vi "Test Constant Waveform Iterate Functions.vi"() -> ()   [LabVIEW 2021]
uses:
  <vilib>/measure/NI_MABase.lvlib
  Source/Constants/Support/WFM/WFM.vi
  Source/Constants/Support/WFM/Const_WFM.lvclass
panel:
  out "Waveform Chart 2":waveform(dbl)(graph)
  out "Waveform Chart":waveform(dbl)(graph)
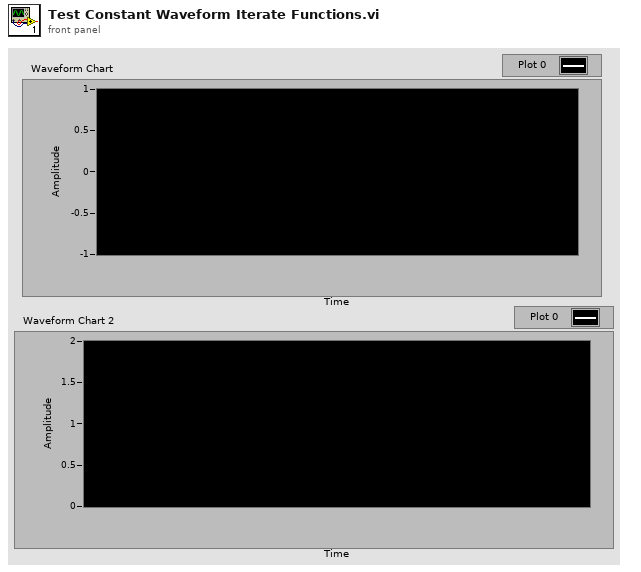
[diagram p1: front panel]
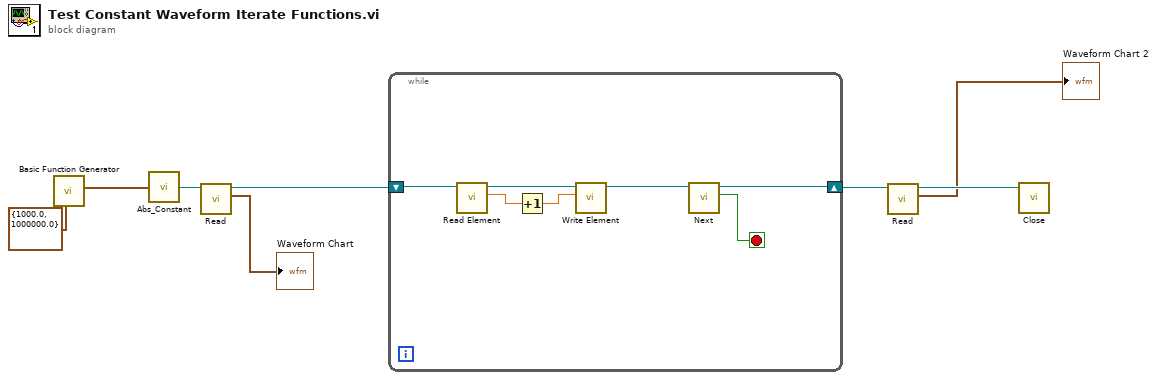
[diagram p0: block diagram]
diagram:
  n1 = call <vilib>:"Basic Function Generator.vi"("sampling info"=cluster{"Fs":dbl, "#s":dbl} {"Fs"=1000.0, "#s"=1000000.0}) -> ("signal out"=w3:waveform(dbl))  [unwired: 8 in, 2 out]
  n2 = call-poly "Abs_Constant.vi"("Value"=w3) -> ("Constant"=w5:refnum<class "Const_WFM.lvclass">)  [unwired: 4 in]
  n3 = call-dynamic "Read.vi"("Const_WFM in"=w5) -> ("Waveform"=→"Waveform Chart":waveform(dbl), "Const_WFM out"=w4:refnum<class "Const_WFM.lvclass">)  [unwired: 8 in, 1 out]
  n4 = while {
    shift-right: [w14] -> w8
    shift-left: w4 -> [w13]
    stop <- w15 stop-if-true
    n5 = call-dynamic "Read Element.vi"("Abs_Waveform in"=w13) -> ("Element"=w10:dbl, "Abs_Waveform out"=w12:refnum<class "Const_WFM.lvclass">)  [unwired: 8 in, 1 out]
    n6 = Increment(x=w10) -> (x+1=w9:dbl)
    n7 = call-dynamic "Write Element.vi"("Element"=w9, "Abs_Waveform in"=w12) -> ("Abs_Waveform out"=w11:refnum<class "Const_WFM.lvclass">)  [unwired: 8 in, 1 out]
    n8 = call-dynamic "Next.vi"("Iterate in"=w11) -> ("Last?"=w15:bool, "Iterate out"=w14:refnum<class "Const_WFM.lvclass">)  [unwired: 8 in, 1 out]
  }
  n9 = call-dynamic "Read.vi"("Const_WFM in"=w8) -> ("Waveform"=→"Waveform Chart 2":waveform(dbl), "Const_WFM out"=w7:refnum<class "Const_WFM.lvclass">)  [unwired: 8 in, 1 out]
  n10 = call-dynamic "Close.vi"("Data in"=w7) -> ()  [unwired: 9 in, 2 out]
